vi "Close Session.vi"(8 "error in":errorcluster, 11 "FPGA Session":T1) -> (0 "error out":errorcluster)   [LabVIEW 2011, in "FlexRIO Host Library (User).lvlib"]
doc: "This start acquisition by switching OFF and ON \"Arm Acquire button\".\nThis VI also starts DMA FIFO."
uses:
  <userlib>/FlexRIO Host Library/FlexRIO Host Library (User).lvlib
  <vilib>/rvi/interface/nirviCloseFPGA/nirviCloseFPGA.xnode
  <vilib>/rvi/interface/nirviMethod/nirviMethod.xnode
  <userlib>/FlexRIO Host Library/FlexRIO Host API/Session/FPGA Session Ref.ctl
  OCT Reference Design/FPGA Bitfiles/OCTDigitizer_FPGABoard_AcquireDatawithout DRAM.lvbitx
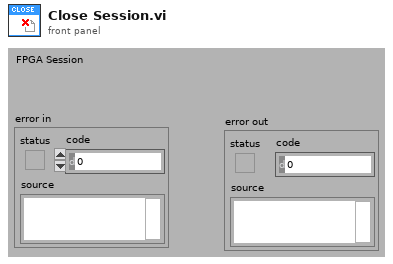
[diagram p1: front panel]
types:
  T1 = typedef "FlexRIO Host Library (User).lvlib/FPGA Session Ref.ctl" = refnum<k20>
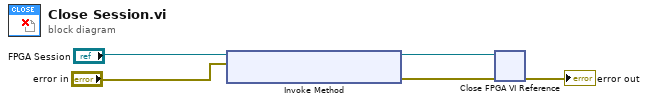
[diagram p0: block diagram]
diagram:
  n1 = xnode "Invoke Method"("FPGA VI Reference In"="FPGA Session", "error in"="error in") -> ("FPGA VI Reference Out"=w2:T1, "error out"=w1:errorcluster)
  n2 = xnode "Close FPGA VI Reference"("FPGA VI Reference In"=w2, "error in"=w1) -> ("error out"=→"error out":errorcluster)
